vi "[GV]_A or M.vi"() -> ()   [LabVIEW 2016]
panel:
  in  "A or M":bool
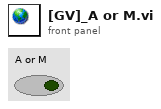
[diagram p1: front panel]
diagram:
